vi "LoadCluster (SubVI).vi"(10 "Datenspeicher":T2={"Fahrzeugdaten"="", "Auto-Pfad"="", "Rolle [Inkr/U]"=0, "Rollenumfang [m]"=0.0, "Rollenträgheit [kgm²]"=0.0, "Zündung [Imp/U]"=0.0, "Getriebe [1:]"=0.0, "Reifenumfang [m] "=0.0, "element"=0.0, "Gl. Mittelwert"=0, "Differenzenquotient"=0, 0, "dT [s]"=0.0, "Strecke [m]"=0.0, "Lufttemperatur [°C]"=0.0, "Mv: n1 [1/min]"=0.0, "Luftdruck [mbar]"=0.0, "nRolle"=[], "nWelle"=[], "AFR"=[], "EGT"=[], "Übersetzung ermitteln aus"=0, "[s]"=0.0, "Mv: M0 [Nm]"=0.0, "Mv: M1 [Nm]"=0.0, "n vom Gas [1/min]"=0.0, "dT ungefiltert [s]"=[], [], "Boolesch"=FALSE, "Serielle Schnittstelle"="COM4", "nKuWe/nRolle 2"=10.0, "v vom Gas [km/h]"=5000.0}, 11 "XML File Path":path caption="XML-Dateipfad") -> (1 "Dateiname":string, 2 "cancelled":bool, 3 "Value":T3)   [LabVIEW 2014]
uses:
  <vilib>/Utility/xml.llb/Read From XML File(string).vi
panel:
  in  "Datenspeicher 2":T1
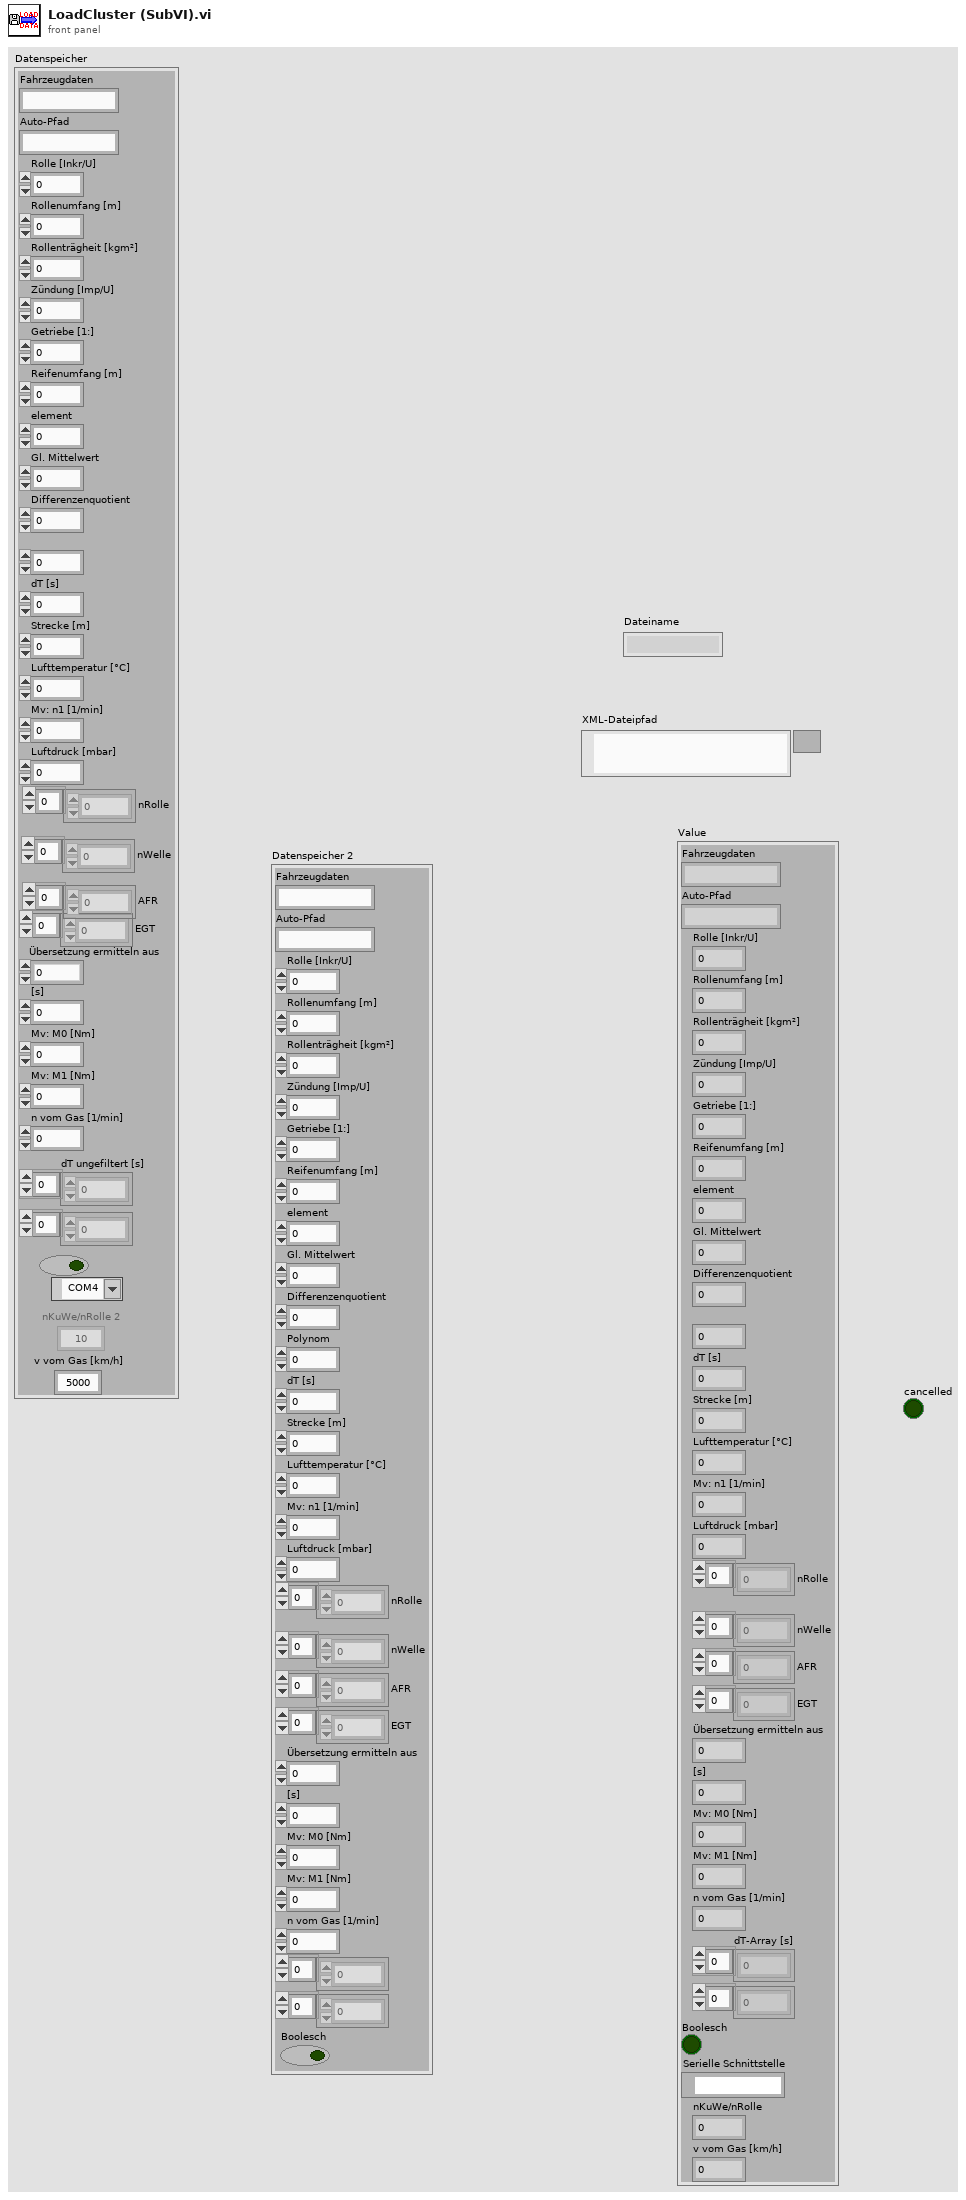
[diagram p1: front panel]
types:
  T1 = cluster{"Fahrzeugdaten":string, "Auto-Pfad":string, "Rolle [Inkr/U]":u16, "Rollenumfang [m]":dbl, "Rollenträgheit [kgm²]":dbl, "Zündung [Imp/U]":dbl, "Getriebe [1:]":dbl, "Reifenumfang [m] ":dbl, "element":dbl, "Gl. Mittelwert":u8, "Differenzenquotient":u8, "Polynom":u8, "dT [s]":dbl, "Strecke [m]":dbl, "Lufttemperatur [°C]":dbl, "Mv: n1 [1/min]":dbl, "Luftdruck [mbar]":dbl, "nRolle":dbl[], "nWelle":dbl[], "AFR":dbl[], "EGT":dbl[], "Übersetzung ermitteln aus":u8, "[s]":dbl, "Mv: M0 [Nm]":dbl, "Mv: M1 [Nm]":dbl, "n vom Gas [1/min]":dbl, dbl[], i32[], "Boolesch":bool}
  T2 = cluster{"Fahrzeugdaten":string, "Auto-Pfad":string, "Rolle [Inkr/U]":u16, "Rollenumfang [m]":dbl, "Rollenträgheit [kgm²]":dbl, "Zündung [Imp/U]":dbl, "Getriebe [1:]":dbl, "Reifenumfang [m] ":dbl, "element":dbl, "Gl. Mittelwert":u8, "Differenzenquotient":u8, u8, "dT [s]":dbl, "Strecke [m]":dbl, "Lufttemperatur [°C]":dbl, "Mv: n1 [1/min]":dbl, "Luftdruck [mbar]":dbl, "nRolle":dbl[], "nWelle":dbl[], "AFR":dbl[], "EGT":dbl[], "Übersetzung ermitteln aus":u8, "[s]":dbl, "Mv: M0 [Nm]":dbl, "Mv: M1 [Nm]":dbl, "n vom Gas [1/min]":dbl, "dT ungefiltert [s]":dbl[], i32[], "Boolesch":bool, "Serielle Schnittstelle":refnum<visa-resource-name>, "nKuWe/nRolle 2":dbl, "v vom Gas [km/h]":dbl}
  T3 = cluster{"Fahrzeugdaten":string, "Auto-Pfad":string, "Rolle [Inkr/U]":u16, "Rollenumfang [m]":dbl, "Rollenträgheit [kgm²]":dbl, "Zündung [Imp/U]":dbl, "Getriebe [1:]":dbl, "Reifenumfang [m] ":dbl, "element":dbl, "Gl. Mittelwert":u8, "Differenzenquotient":u8, u8, "dT [s]":dbl, "Strecke [m]":dbl, "Lufttemperatur [°C]":dbl, "Mv: n1 [1/min]":dbl, "Luftdruck [mbar]":dbl, "nRolle":dbl[], "nWelle":dbl[], "AFR":dbl[], "EGT":dbl[], "Übersetzung ermitteln aus":u8, "[s]":dbl, "Mv: M0 [Nm]":dbl, "Mv: M1 [Nm]":dbl, "n vom Gas [1/min]":dbl, "dT-Array [s]":dbl[], i32[], "Boolesch":bool, "Serielle Schnittstelle":refnum<visa-resource-name>, "nKuWe/nRolle":dbl, "v vom Gas [km/h]":dbl}
  T4 = cluster{"Fahrzeugdaten":string, "Auto-Pfad":string, "Rolle [Inkr/U]":u16, "Rollenumfang [m]":dbl, "Rollenträgheit [kgm²]":dbl, "Zündung [Imp/U]":dbl, "Getriebe [1:]":dbl, "Reifenumfang [m] ":dbl, "element":dbl, "Gl. Mittelwert":u8, "Differenzenquotient":u8, "Live Aktualisierungs-Geschwindigkeit":u8, "dT [s]":dbl, "Strecke [m]":dbl, "Lufttemperatur [°C]":dbl, "Mv: n1 [1/min]":dbl, "Luftdruck [mbar]":dbl, "nRolle":dbl[], "nWelle":dbl[], "AFR":dbl[], "EGT":dbl[], "Übersetzung ermitteln aus":u8, "[s]":dbl, "Mv: M0 [Nm]":dbl, "Mv: M1 [Nm]":dbl, "n vom Gas [1/min]":dbl, "dT-Array [s]":dbl[], i32[], "Boolesch":bool, "Serielle Schnittstelle":refnum<visa-resource-name>, "nKuWe/nRolle":dbl}
  T5 = cluster{"Fahrzeugdaten":string, "Auto-Pfad":string, "Rolle [Inkr/U]":u16, "Rollenumfang [m]":dbl, "Rollenträgheit [kgm²]":dbl, "Zündung [Imp/U]":dbl, "Getriebe [1:]":dbl, "Reifenumfang [m] ":dbl, "element":dbl, "Gl. Mittelwert":u8, "Differenzenquotient":u8, "Live Aktualisierungs-Geschwindigkeit":u8, "dT[s]":dbl, "Strecke [m]":dbl, "Lufttemperatur [°C]":dbl, "Mv: n1 [1/min]":dbl, "Luftdruck [mbar]":dbl, "nRolle":dbl[], "nWelle":dbl[], "AFR":dbl[], "EGT":dbl[], "Übersetzung ermitteln aus":u8, "[s]":dbl, "Mv: M0 [Nm]":dbl, "Mv: M1 [Nm]":dbl, "n vom Gas [1/min]":dbl, dbl[], i32[], "Boolesch":bool, "Serielle Schnittstelle":refnum<visa-resource-name>}
  T6 = cluster{"Fahrzeugdaten":string, "Auto-Pfad":string, "Rolle [Inkr/U]":u16, "Rollenumfang [m]":dbl, "Rollenträgheit [kgm²]":dbl, "Zündung [Imp/U]":dbl, "Getriebe [1:]":dbl, "Reifenumfang [m] ":dbl, "element":dbl, "Gl. Mittelwert":u8, "Differenzenquotient":u8, "Live Aktualisierungs-Geschwindigkeit":u8, "dT [s]":dbl, "Strecke [m]":dbl, "Lufttemperatur [°C]":dbl, "Mv: n1 [1/min]":dbl, "Luftdruck [mbar]":dbl, "nRolle":dbl[], "nWelle":dbl[], "AFR":dbl[], "EGT":dbl[], "Übersetzung ermitteln aus":u8, "[s]":dbl, "Mv: M0 [Nm]":dbl, "Mv: M1 [Nm]":dbl, "n vom Gas [1/min]":dbl, "dT-Array [s]":dbl[], i32[], "Boolesch":bool, "Serielle Schnittstelle":refnum<visa-resource-name>, "nKuWe/nRolle":dbl, "v vom Gas [km/h]":dbl}
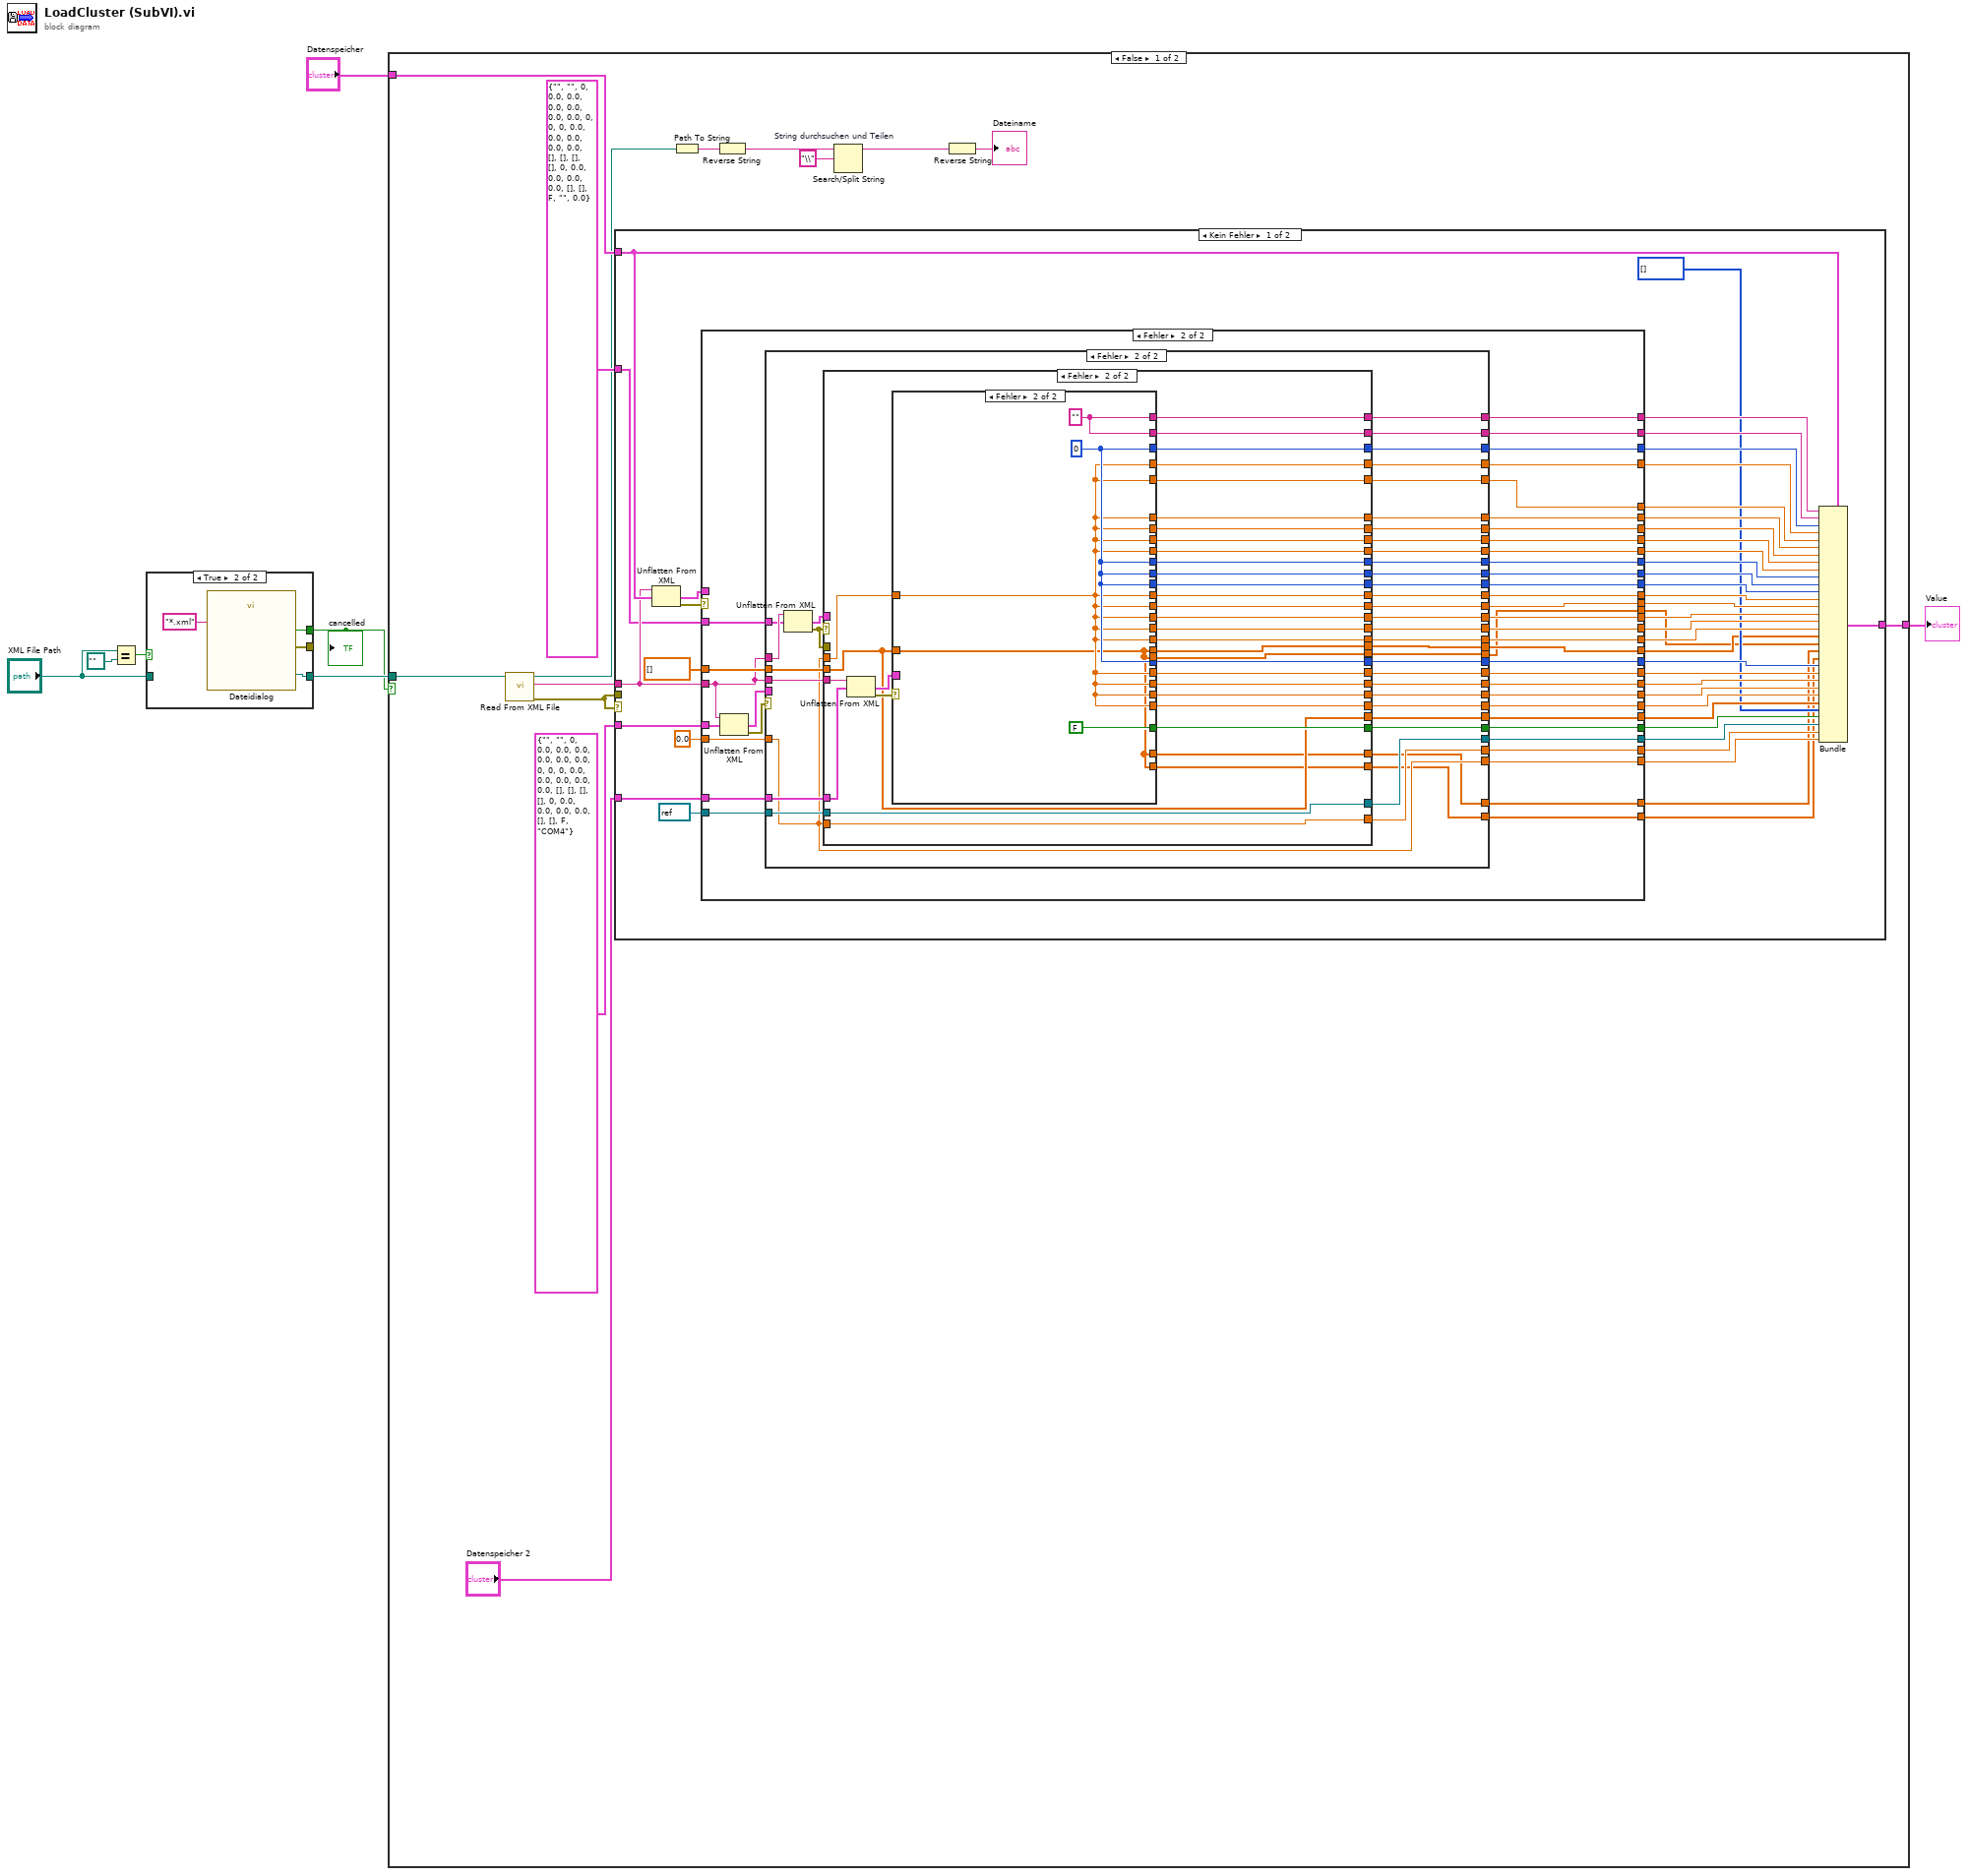
[diagram p0: block diagram]
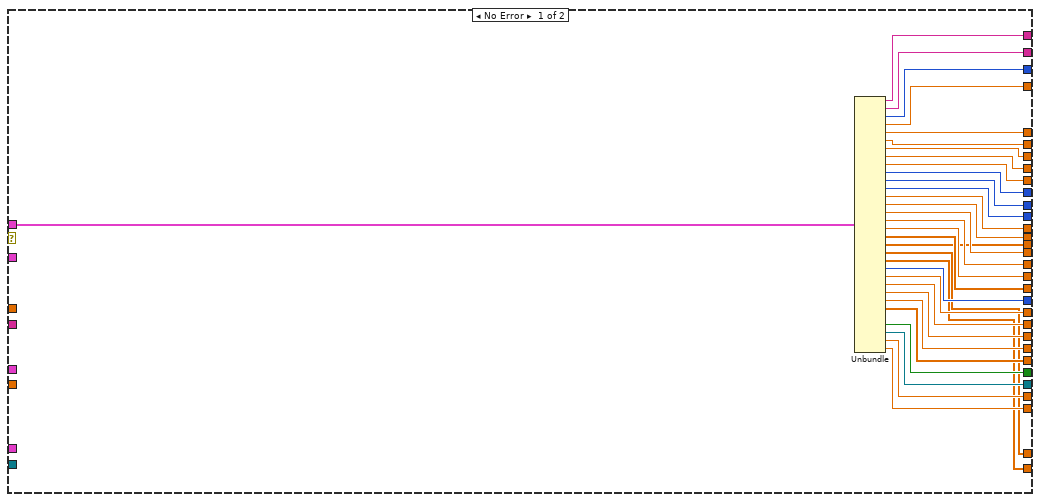
[diagram p2: hidden frame]
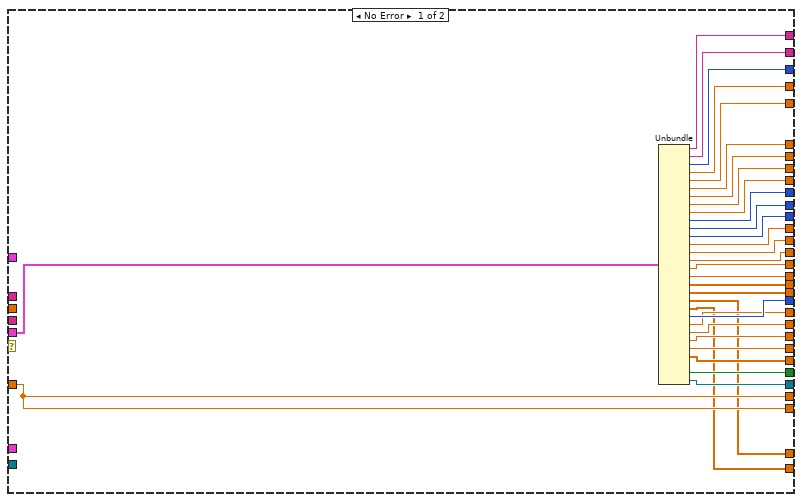
[diagram p3: hidden frame]
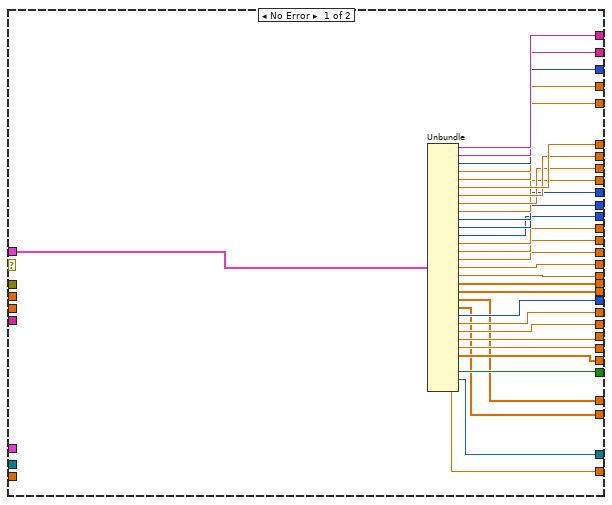
[diagram p4: hidden frame]
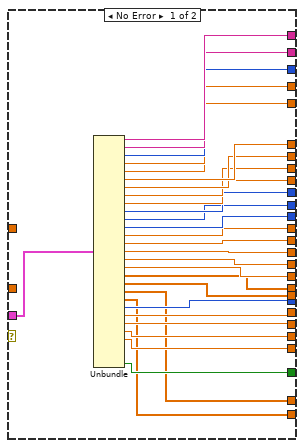
[diagram p5: hidden frame]
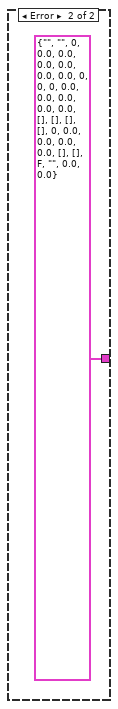
[diagram p6: hidden frame]
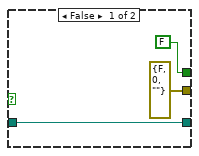
[diagram p8: hidden frame]
diagram:
  n1 = Equal?(x="XML File Path", y=path "") -> (x = y?=w6:bool)
  n2 = case shown="True" w6 {
    tunnel: [w10 w14] -> w5
    tunnel: "XML File Path" -> [w10 _]
    tunnel: [FALSE ("cancelled") w12] -> w3
    tunnel: [errorcluster {"status"=FALSE, "code"=0, "source"=""} ("error out") w11] -> _
    frame False {
    }
    frame True {
      n3 = call "Dateidialog"("pattern (all files)"="*.xml") -> ("selected path"=w14:path, "cancelled"=w12:bool, "error out"=w11:errorcluster)  [unwired: 11 in, 1 out]
    }
  }
  "cancelled" <- w3
  n4 = case shown="False" w3 {
    tunnel: w5 -> [w28 _]
    tunnel: [w22 w314] -> w2
    tunnel: "Datenspeicher" -> [w21 w314]
    frame False {
      n5 = call-poly <vilib>:"Read From XML File.vi"("XML File Path"=w28) -> ("error out"=w23:errorcluster, "XML Elements"=w27:string, "XML File Path(duplicate)"=w17:path)  [unwired: 8 in]
      n6 = case shown="Kein Fehler" w23 {
        tunnel: w27 -> [w50 _]
        tunnel: w21 -> [w71 _]
        tunnel: w23 -> [_ _]
        tunnel: T5 {"Fahrzeugdaten"="", "Auto-Pfad"="", "Rolle [Inkr/U]"=0, "Rollenumfang [m]"=0.0, "Rollenträgheit [kgm²]"=0.0, "Zündung [Imp/U]"=0.0, "Getriebe [1:]"=0.0, "Reifenumfang [m] "=0.0, "element"=0.0, "Gl. Mittelwert"=0, "Differenzenquotient"=0, "Live Aktualisierungs-Geschwindigkeit"=0, "dT[s]"=0.0, "Strecke [m]"=0.0, "Lufttemperatur [°C]"=0.0, "Mv: n1 [1/min]"=0.0, "Luftdruck [mbar]"=0.0, "nRolle"=[], "nWelle"=[], "AFR"=[], "EGT"=[], "Übersetzung ermitteln aus"=0, "[s]"=0.0, "Mv: M0 [Nm]"=0.0, "Mv: M1 [Nm]"=0.0, "n vom Gas [1/min]"=0.0, [], [], "Boolesch"=FALSE, "Serielle Schnittstelle"="COM4"} ("Datenspeicher") -> [w51 _]
        tunnel: "Datenspeicher 2" -> [w49 _]
        tunnel: T4 {"Fahrzeugdaten"="", "Auto-Pfad"="", "Rolle [Inkr/U]"=0, "Rollenumfang [m]"=0.0, "Rollenträgheit [kgm²]"=0.0, "Zündung [Imp/U]"=0.0, "Getriebe [1:]"=0.0, "Reifenumfang [m] "=0.0, "element"=0.0, "Gl. Mittelwert"=0, "Differenzenquotient"=0, "Live Aktualisierungs-Geschwindigkeit"=0, "dT [s]"=0.0, "Strecke [m]"=0.0, "Lufttemperatur [°C]"=0.0, "Mv: n1 [1/min]"=0.0, "Luftdruck [mbar]"=0.0, "nRolle"=[], "nWelle"=[], "AFR"=[], "EGT"=[], "Übersetzung ermitteln aus"=0, "[s]"=0.0, "Mv: M0 [Nm]"=0.0, "Mv: M1 [Nm]"=0.0, "n vom Gas [1/min]"=0.0, "dT-Array [s]"=[], [], "Boolesch"=FALSE, "Serielle Schnittstelle"="", "nKuWe/nRolle"=0.0} ("Speicher V1.0.3") -> [w45 _]
        tunnel: [w44 T6 {"Fahrzeugdaten"="", "Auto-Pfad"="", "Rolle [Inkr/U]"=0, "Rollenumfang [m]"=0.0, "Rollenträgheit [kgm²]"=0.0, "Zündung [Imp/U]"=0.0, "Getriebe [1:]"=0.0, "Reifenumfang [m] "=0.0, "element"=0.0, "Gl. Mittelwert"=0, "Differenzenquotient"=0, "Live Aktualisierungs-Geschwindigkeit"=0, "dT [s]"=0.0, "Strecke [m]"=0.0, "Lufttemperatur [°C]"=0.0, "Mv: n1 [1/min]"=0.0, "Luftdruck [mbar]"=0.0, "nRolle"=[], "nWelle"=[], "AFR"=[], "EGT"=[], "Übersetzung ermitteln aus"=0, "[s]"=0.0, "Mv: M0 [Nm]"=0.0, "Mv: M1 [Nm]"=0.0, "n vom Gas [1/min]"=0.0, "dT-Array [s]"=[], [], "Boolesch"=FALSE, "Serielle Schnittstelle"="", "nKuWe/nRolle"=0.0, "v vom Gas [km/h]"=0.0} ("Speicher V2.0.5")] -> w22
        frame No Error {
          n7 = Unflatten From XML(xml string=w50, type=w71) -> (value=w52:T2, error out=w53:errorcluster)  [unwired: 1 in]
          n8 = case shown="Fehler" w53 {
            tunnel: w52 -> [w103 _]
            tunnel: [w102 w141] -> w70
            tunnel: [w101 w140] -> w69
            tunnel: [w100 w139] -> w68
            tunnel: [w99 w138] -> w67
            tunnel: [w98 w137] -> w66
            tunnel: [w97 w136] -> w65
            tunnel: [w96 w135] -> w64
            tunnel: [w95 w134] -> w63
            tunnel: [w94 w133] -> w62
            tunnel: [w93 w132] -> w61
            tunnel: [w92 w131] -> w60
            tunnel: [w91 w130] -> w59
            tunnel: [w90 w129] -> w58
            tunnel: [w89 w128] -> w57
            tunnel: [w88 w127] -> w56
            tunnel: [w87 w126] -> w55
            tunnel: [w86 w125] -> w54
            tunnel: [w85 w124] -> w32
            tunnel: [w80 w123] -> w35
            tunnel: [w79 w122] -> w34
            tunnel: [w78 w121] -> w36
            tunnel: [w77 w120] -> w37
            tunnel: [w76 w119] -> w38
            tunnel: [w75 w116] -> w39
            tunnel: [w81 w118] -> w40
            tunnel: [w82 w117] -> w41
            tunnel: [w83 w115] -> w42
            tunnel: [w84 w114] -> w43
            tunnel: w51 -> [_ w143]
            tunnel: w50 -> [_ w108]
            tunnel: w49 -> [_ w112]
            tunnel: dbl[] [] ("dT-Array [s]") -> [_ w111]
            tunnel: 0.0 ("nKuWe/nRolle") -> [_ w110]
            tunnel: refnum<visa-resource-name> refnum ("Serielle Schnittstelle") -> [_ w109]
            tunnel: w45 -> [_ w107]
            tunnel: [w74 w106] -> w31
            tunnel: [w73 w105] -> w30
            tunnel: [w72 w104] -> w29
            frame No Error {
              n9 = Unbundle(w103) -> ("Fahrzeugdaten"=w102:string, "Auto-Pfad"=w101:string, "Rolle [Inkr/U]"=w100:u16, "Rollenumfang [m]"=w99:dbl, "Rollenträgheit [kgm²]"=w98:dbl, "Zündung [Imp/U]"=w97:dbl, "Getriebe [1:]"=w96:dbl, "Reifenumfang [m]"=w95:dbl, "element"=w94:dbl, "Gl. Mittelwert"=w93:u8, "Differenzenquotient"=w92:u8, w91:u8, "dT [s]"=w90:dbl, "Strecke [m]"=w89:dbl, "Lufttemperatur [°C]"=w88:dbl, "Mv: n1 [1/min]"=w87:dbl, "Luftdruck [mbar]"=w86:dbl, "nRolle"=w85:dbl[], "nWelle"=w74:dbl[], "AFR"=w73:dbl[], "EGT"=w72:dbl[], "Übersetzung ermitteln aus"=w80:u8, "[s]"=w79:dbl, "Mv: M0 [Nm]"=w78:dbl, "Mv: M1 [Nm]"=w77:dbl, "n vom Gas [1/min]"=w76:dbl, "dT ungefiltert [s]"=w75:dbl[], "Boolesch"=w81:bool, "Serielle Schnittstelle"=w82:refnum<visa-resource-name>, "nKuWe/nRolle 2"=w83:dbl, "v vom Gas [km/h]"=w84:dbl)  [unwired: 1 out]
            }
            frame Error {
              n10 = Unflatten From XML(xml string=w108, type=w143) -> (value=w142:T5, error out=w113:errorcluster)  [unwired: 1 in]
              n11 = case shown="Fehler" w113 {
                tunnel: w142 -> [w174 _]
                tunnel: [w173 w211] -> w141
                tunnel: [w172 w210] -> w140
                tunnel: [w171 w209] -> w139
                tunnel: [w170 w208] -> w138
                tunnel: [w169 w207] -> w137
                tunnel: [w168 w206] -> w136
                tunnel: [w167 w205] -> w135
                tunnel: [w166 w204] -> w134
                tunnel: [w165 w203] -> w133
                tunnel: [w164 w202] -> w132
                tunnel: [w163 w201] -> w131
                tunnel: [w162 w200] -> w130
                tunnel: [w161 w199] -> w129
                tunnel: [w160 w198] -> w128
                tunnel: [w159 w197] -> w127
                tunnel: [w158 w196] -> w126
                tunnel: [w157 w195] -> w125
                tunnel: [w156 w194] -> w124
                tunnel: [w154 w193] -> w123
                tunnel: [w153 w192] -> w122
                tunnel: [w152 w191] -> w121
                tunnel: [w151 w190] -> w120
                tunnel: [w150 w189] -> w119
                tunnel: [w148 w188] -> w118
                tunnel: [w147 w182] -> w117
                tunnel: [w149 w178] -> w116
                tunnel: [w155 w180] -> w115
                tunnel: [w155 w179] -> w114
                tunnel: w108 -> [_ w213]
                tunnel: w112 -> [_ w212]
                tunnel: w111 -> [_ w185]
                tunnel: w110 -> [w155 w179]
                tunnel: w109 -> [_ w181]
                tunnel: w108 -> [_ w187]
                tunnel: w107 -> [_ w186]
                tunnel: [w146 w177] -> w106
                tunnel: [w145 w176] -> w105
                tunnel: [w144 w175] -> w104
                frame No Error {
                  n12 = Unbundle(w174) -> ("Fahrzeugdaten"=w173:string, "Auto-Pfad"=w172:string, "Rolle [Inkr/U]"=w171:u16, "Rollenumfang [m]"=w170:dbl, "Rollenträgheit [kgm²]"=w169:dbl, "Zündung [Imp/U]"=w168:dbl, "Getriebe [1:]"=w167:dbl, "Reifenumfang [m]"=w166:dbl, "element"=w165:dbl, "Gl. Mittelwert"=w164:u8, "Differenzenquotient"=w163:u8, "Live Aktualisierungs-Geschwindigkeit"=w162:u8, "dT[s]"=w161:dbl, "Strecke [m]"=w160:dbl, "Lufttemperatur [°C]"=w159:dbl, "Mv: n1 [1/min]"=w158:dbl, "Luftdruck [mbar]"=w157:dbl, "nRolle"=w156:dbl[], "nWelle"=w146:dbl[], "AFR"=w145:dbl[], "EGT"=w144:dbl[], "Übersetzung ermitteln aus"=w154:u8, "[s]"=w153:dbl, "Mv: M0 [Nm]"=w152:dbl, "Mv: M1 [Nm]"=w151:dbl, "n vom Gas [1/min]"=w150:dbl, w149:dbl[], "Boolesch"=w148:bool, "Serielle Schnittstelle"=w147:refnum<visa-resource-name>)  [unwired: 1 out]
                }
                frame Error {
                  n13 = Unflatten From XML(xml string=w187, type=w186) -> (value=w183:T4, error out=w184:errorcluster)  [unwired: 1 in]
                  n14 = case shown="Fehler" w184 {
                    tunnel: w213 -> [_ w279]
                    tunnel: w212 -> [_ w278]
                    tunnel: [w243 w276] -> w211
                    tunnel: [w242 w275] -> w210
                    tunnel: [w241 w274] -> w209
                    tunnel: [w240 w273] -> w208
                    tunnel: [w239 w272] -> w207
                    tunnel: [w238 w271] -> w206
                    tunnel: [w237 w270] -> w205
                    tunnel: [w236 w269] -> w204
                    tunnel: [w235 w268] -> w203
                    tunnel: [w234 w267] -> w202
                    tunnel: [w233 w266] -> w201
                    tunnel: [w232 w265] -> w200
                    tunnel: [w231 w264] -> w199
                    tunnel: [w230 w263] -> w198
                    tunnel: [w229 w262] -> w197
                    tunnel: [w228 w261] -> w196
                    tunnel: [w227 w260] -> w195
                    tunnel: [w226 w259] -> w194
                    tunnel: [w225 w258] -> w193
                    tunnel: [w224 w257] -> w192
                    tunnel: [w223 w256] -> w191
                    tunnel: [w222 w255] -> w190
                    tunnel: [w218 w254] -> w189
                    tunnel: [w219 w253] -> w188
                    tunnel: w184 -> [_ _]
                    tunnel: w179 -> [_ w251]
                    tunnel: w185 -> [_ w248]
                    tunnel: w183 -> [w244 _]
                    tunnel: [w221 w250] -> w182
                    tunnel: w181 -> [_ w250]
                    tunnel: [w220 w249] -> w180
                    tunnel: w179 -> [_ w249]
                    tunnel: [w217 w248] -> w178
                    tunnel: [w216 w247] -> w177
                    tunnel: [w215 w246] -> w176
                    tunnel: [w214 w245] -> w175
                    frame No Error {
                      n15 = Unbundle(w244) -> ("Fahrzeugdaten"=w243:string, "Auto-Pfad"=w242:string, "Rolle [Inkr/U]"=w241:u16, "Rollenumfang [m]"=w240:dbl, "Rollenträgheit [kgm²]"=w239:dbl, "Zündung [Imp/U]"=w238:dbl, "Getriebe [1:]"=w237:dbl, "Reifenumfang [m]"=w236:dbl, "element"=w235:dbl, "Gl. Mittelwert"=w234:u8, "Differenzenquotient"=w233:u8, "Live Aktualisierungs-Geschwindigkeit"=w232:u8, "dT [s]"=w231:dbl, "Strecke [m]"=w230:dbl, "Lufttemperatur [°C]"=w229:dbl, "Mv: n1 [1/min]"=w228:dbl, "Luftdruck [mbar]"=w227:dbl, "nRolle"=w226:dbl[], "nWelle"=w216:dbl[], "AFR"=w215:dbl[], "EGT"=w214:dbl[], "Übersetzung ermitteln aus"=w225:u8, "[s]"=w224:dbl, "Mv: M0 [Nm]"=w223:dbl, "Mv: M1 [Nm]"=w222:dbl, "n vom Gas [1/min]"=w218:dbl, "dT-Array [s]"=w217:dbl[], "Boolesch"=w219:bool, "Serielle Schnittstelle"=w221:refnum<visa-resource-name>, "nKuWe/nRolle"=w220:dbl)  [unwired: 1 out]
                    }
                    frame Error {
                      n16 = Unflatten From XML(xml string=w279, type=w278) -> (value=w277:T1, error out=w252:errorcluster)  [unwired: 1 in]
                      n17 = case shown="Fehler" w252 {
                        tunnel: w277 -> [w307 _]
                        tunnel: [w306 w312] -> w276
                        tunnel: [w305 w312] -> w275
                        tunnel: [w304 w311] -> w274
                        tunnel: [w303 w309] -> w273
                        tunnel: [w302 w309] -> w272
                        tunnel: [w301 w309] -> w271
                        tunnel: [w300 w309] -> w270
                        tunnel: [w299 w309] -> w269
                        tunnel: [w298 w309] -> w268
                        tunnel: [w297 w311] -> w267
                        tunnel: [w296 w311] -> w266
                        tunnel: [w295 w311] -> w265
                        tunnel: [w294 w309] -> w264
                        tunnel: [w293 w309] -> w263
                        tunnel: [w292 w309] -> w262
                        tunnel: [w291 w309] -> w261
                        tunnel: [w290 w309] -> w260
                        tunnel: [w289 w308] -> w259
                        tunnel: [w287 w311] -> w258
                        tunnel: [w286 w309] -> w257
                        tunnel: [w285 w309] -> w256
                        tunnel: [w284 w309] -> w255
                        tunnel: [w283 w309] -> w254
                        tunnel: [w288 FALSE ("Boolesch")] -> w253
                        tunnel: w251 -> [_ w309]
                        tunnel: w248 -> [_ w308]
                        tunnel: [w282 w308] -> w247
                        tunnel: [w281 w308] -> w246
                        tunnel: [w280 w308] -> w245
                        frame No Error {
                          n18 = Unbundle(w307) -> ("Fahrzeugdaten"=w306:string, "Auto-Pfad"=w305:string, "Rolle [Inkr/U]"=w304:u16, "Rollenumfang [m]"=w303:dbl, "Rollenträgheit [kgm²]"=w302:dbl, "Zündung [Imp/U]"=w301:dbl, "Getriebe [1:]"=w300:dbl, "Reifenumfang [m]"=w299:dbl, "element"=w298:dbl, "Gl. Mittelwert"=w297:u8, "Differenzenquotient"=w296:u8, "Polynom"=w295:u8, "dT [s]"=w294:dbl, "Strecke [m]"=w293:dbl, "Lufttemperatur [°C]"=w292:dbl, "Mv: n1 [1/min]"=w291:dbl, "Luftdruck [mbar]"=w290:dbl, "nRolle"=w289:dbl[], "nWelle"=w282:dbl[], "AFR"=w281:dbl[], "EGT"=w280:dbl[], "Übersetzung ermitteln aus"=w287:u8, "[s]"=w286:dbl, "Mv: M0 [Nm]"=w285:dbl, "Mv: M1 [Nm]"=w284:dbl, "n vom Gas [1/min]"=w283:dbl, "Boolesch"=w288:bool)  [unwired: 2 out]
                        }
                        frame Error {
                          w311 = u16 0 ("Rolle [Inkr/U]")
                          w312 = "" ("Fahrzeugdaten")
                        }
                      }
                    }
                  }
                }
              }
            }
          }
          n19 = Bundle(cluster=w71, "Fahrzeugdaten"=w70, "Auto-Pfad"=w69, "Rolle [Inkr/U]"=w68, "Rollenumfang [m]"=w67, "Rollenträgheit [kgm²]"=w66, "Zündung [Imp/U]"=w65, "Getriebe [1:]"=w64, "Reifenumfang [m]"=w63, "element"=w62, "Gl. Mittelwert"=w61, "Differenzenquotient"=w60, w59, "dT [s]"=w58, "Strecke [m]"=w57, "Lufttemperatur [°C]"=w56, "Mv: n1 [1/min]"=w55, "Luftdruck [mbar]"=w54, "nRolle"=w32, "nWelle"=w31, "AFR"=w30, "EGT"=w29, "Übersetzung ermitteln aus"=w35, "[s]"=w34, "Mv: M0 [Nm]"=w36, "Mv: M1 [Nm]"=w37, "n vom Gas [1/min]"=w38, "dT ungefiltert [s]"=w39, i32[] [], "Boolesch"=w40, "Serielle Schnittstelle"=w41, "nKuWe/nRolle 2"=w42, "v vom Gas [km/h]"=w43) -> (w44:T2)
        }
        frame Error {
        }
      }
      n20 = Path To String(path=w17) -> (string=w18:string)
      n21 = Reverse String(1:w18) -> (0:w16:string)
      n22 = Search/Split String "String durchsuchen und Teilen"(string=w16, search string/char (-)="\\") -> (substring before match=w19:string)  [unwired: 1 in, 2 out]
      n23 = Reverse String(1:w19) -> (0:→"Dateiname":string)
    }
    frame True {
    }
  }
  "Value" <- w2
